vi "0-Load Boat Icon.vi"() -> (0 "Overlay References Out":T1)   [LabVIEW 2011]
doc: "Loads the boat icon for use on the map. Also, replaces all the black pixels with transparent pixels."
uses:
  0 Typedefs/Overlay References.ctl
  <vilib>/vision/Image Controls.llb/IMAQ Image.ctl
panel:
  out "appended sail icon path":path
  out "Image":T2(plugin-control)
  out "appended boat icon path":path
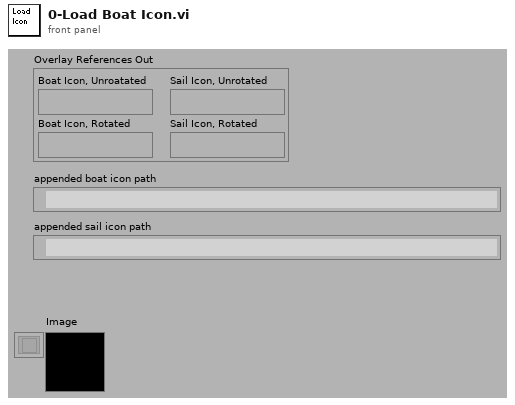
[diagram p1: front panel]
types:
  T1 = typedef "Overlay References.ctl" = cluster{"Boat Icon, Unroatated":T2, "Boat Icon, Rotated":T2, "Sail Icon, Unrotated":T2, "Sail Icon, Rotated":T2}
  T2 = typedef "IMAQ Image.ctl" = refnum<image>
  T3 = typedef "Image Type" = u32
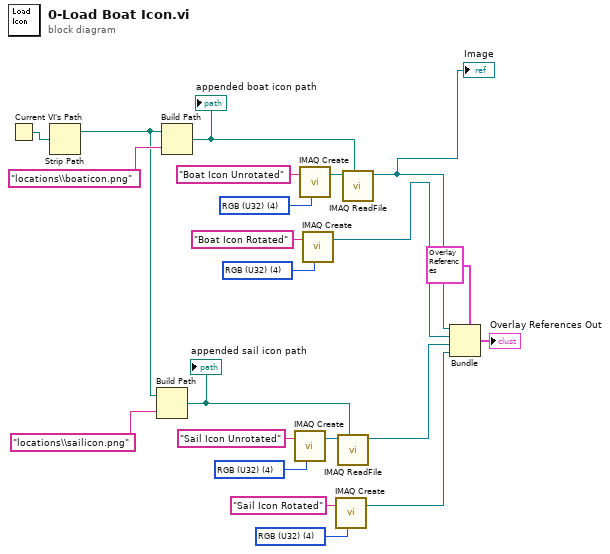
[diagram p0: block diagram]
diagram:
  w8 = T3 4 items=["Grayscale (U8)", "Grayscale (I16)", "Grayscale (SGL)", "Complex (CSG)", "RGB (U32)", "HSL (U32)", "RGB (U64)", "Grayscale (U16)"] ("Image Type")
  w10 = T3 4 items=["Grayscale (U8)", "Grayscale (I16)", "Grayscale (SGL)", "Complex (CSG)", "RGB (U32)", "HSL (U32)", "RGB (U64)", "Grayscale (U16)"] ("Image Type")
  w15 = T3 4 items=["Grayscale (U8)", "Grayscale (I16)", "Grayscale (SGL)", "Complex (CSG)", "RGB (U32)", "HSL (U32)", "RGB (U64)", "Grayscale (U16)"] ("Image Type")
  w22 = T3 4 items=["Grayscale (U8)", "Grayscale (I16)", "Grayscale (SGL)", "Complex (CSG)", "RGB (U32)", "HSL (U32)", "RGB (U64)", "Grayscale (U16)"] ("Image Type")
  n1 = Current VI's Path() -> (path=w19:path)
  n2 = Strip Path(path=w19) -> (stripped path=w9:path)  [unwired: 1 out]
  n3 = Build Path(base path=w9, name or relative path="locations\\sailicon.png") -> (appended path=w14:path)
  "appended sail icon path" <- w14
  n4 = Build Path(base path=w9, name or relative path="locations\\boaticon.png") -> (appended path=w17:path)
  "appended boat icon path" <- w17
  n5 = call "IMAQ Create"("Image Name"="Sail Icon Unrotated", "Image Type"=w10) -> ("New Image"=w12:T2)  [unwired: 2 in, 2 out]
  n6 = call "IMAQ Create"("Image Name"="Boat Icon Unrotated", "Image Type"=w22) -> ("New Image"=w20:T2)  [unwired: 2 in, 2 out]
  n7 = call "IMAQ Create"("Image Name"="Boat Icon Rotated", "Image Type"=w15) -> ("New Image"=w4:T2)  [unwired: 2 in, 2 out]
  n8 = call "IMAQ Create"("Image Name"="Sail Icon Rotated", "Image Type"=w8) -> ("New Image"=w6:T2)  [unwired: 2 in, 2 out]
  n9 = call "IMAQ ReadFile"("File Path"=w14, "Image"=w12) -> ("Image Out"=w5:T2)  [unwired: 3 in, 6 out]
  n10 = call "IMAQ ReadFile"("File Path"=w17, "Image"=w20) -> ("Image Out"=w3:T2)  [unwired: 3 in, 6 out]
  "Image" <- w3
  n11 = Bundle(cluster=T1 {"Boat Icon, Unroatated"=refnum, "Boat Icon, Rotated"=refnum, "Sail Icon, Unrotated"=refnum, "Sail Icon, Rotated"=refnum} ("Overlay References Out 2"), "Boat Icon, Unroatated"=w3, "Boat Icon, Rotated"=w4, "Sail Icon, Unrotated"=w5, "Sail Icon, Rotated"=w6) -> (→"Overlay References Out":T1)
